vi "set_params.vi"(8 "error in (no error)":errorcluster caption="entrée d'erreur (pas d'erreur)", 11 "GradientBoostingClassifier.lvclass 2":refnum<class "GradientBoostingClassifier.lvclass">) -> (0 "error out":errorcluster caption="sortie d'erreur", 3 "GradientBoostingClassifier.lvclass":refnum<class "GradientBoostingClassifier.lvclass">)   [LabVIEW 2020, in "GradientBoostingClassifier.lvclass"]
uses:
  GradientBoostingClassifier.lvclass
  GradientBoostingClassifier.lvclass/GradientBoostingClassifier.ctl
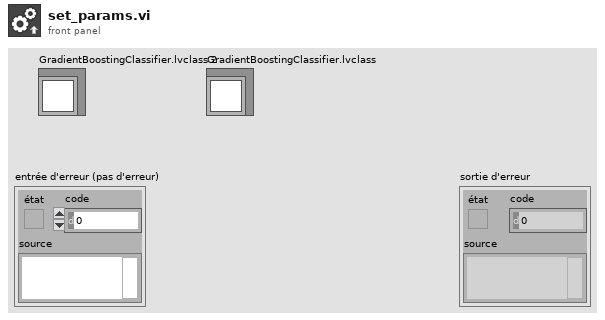
[diagram p1: front panel]
types:
  T1 = typedef "gradient_boosting_classifier_params.ctl" = cluster{"loss":string, "learning_rate":dbl, "n_estimators":dbl, "subsample":dbl, "criterion":string, "min_samples_split":dbl, "min_samples_leaf":dbl, "min_weight_fraction_leaf":dbl, "max_depth":cluster{"max_depth_type":string, "max_depth_int":dbl}, "min_impurity_decrease":dbl, "init":string, "random_state":dbl, "max_features":cluster{"max_features_type":string, "max_features_float":dbl, "max_features_int":dbl}, "verbose":dbl, "max_leaf_nodes":cluster{"max_leaf_nodes_type":string, "max_leaf_nodes_int":dbl}, "warm_start":bool, "validation_fraction":dbl, "n_iter_no_change":cluster{"n_iter_no_change_type":string, "n_iter_no_change_int":dbl}, "tol":dbl, "ccp_alpha":dbl}
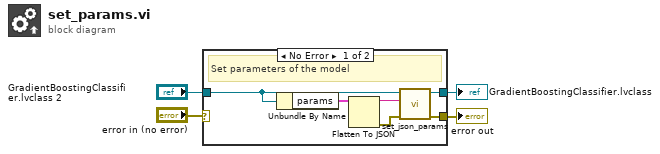
[diagram p0: block diagram]
diagram:
  n1 = case shown="No Error" "error in (no error)" {
    selector: "error in (no error)" -> [_ w12]
    tunnel: [w7 w12] -> w3
    tunnel: [w8 w11] -> w1
    tunnel: "GradientBoostingClassifier.lvclass 2" -> [w5 w11]
    frame No Error {
      # "Set parameters of the model"
      n2 = Unbundle By Name(w5) -> ("params"=w10:T1)
      n3 = Flatten To JSON(anything=w10) -> (JSON string=w9:string, 11:w6:errorcluster)  [unwired: 2 in]
      n4 = call-dynamic "set_json_params.vi"("error in (no error)"=w6, "params"=w9, "Model en entrée"=w5) -> ("error out"=w7:errorcluster, "Model en sortie"=w8:refnum<class "GradientBoostingClassifier.lvclass">)  [unwired: 7 in]
    }
    frame Error {
    }
  }
  "error out" <- w3
  "GradientBoostingClassifier.lvclass" <- w1
